vi "Configure Unmask.vi"(8 "error in (no error)":errorcluster, 10 "Unmask Variable (NONE)":string(combo)="NONE", 11 "VISA resource name":refnum<visa-resource-name>) -> (0 "error out":errorcluster, 3 "VISA resource name out":refnum<visa-resource-name>)   [LabVIEW 2021, in "Sorensen M9A Series.lvlib"]
doc: "This VI enables the supply's operating conditions for fault occurence. The possible values are:\nCV (constant voltage)\nCC (constant current)\nOV (overvoltage protection)\nOT (overtemperature protection)\nSD (shutdown)\nFOLD (foldback)\nNONE (all conditions enabled)\nALL (all conditions disabled)\nThe power supply's default value is NONE."
uses:
  Sorensen M9A Series.lvlib
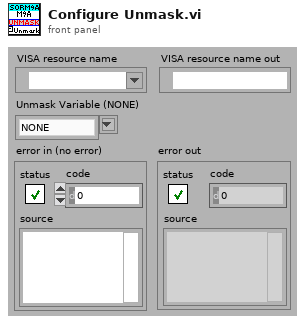
[diagram p1: front panel]
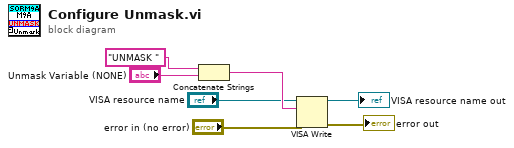
[diagram p0: block diagram]
diagram:
  n1 = Concatenate Strings("UNMASK ", "Unmask Variable (NONE)") -> (w4:string)
  n2 = VISA Write(VISA resource name="VISA resource name", write buffer=w4, error in (no error)="error in (no error)") -> (VISA resource name out=→"VISA resource name out":refnum<visa-resource-name>, error out=→"error out":errorcluster)  [unwired: 1 out]
